vi "Request Events FG.vi"(7 "Action (Get)":enum16{"Initialize", "Get", "Destroy"}(ring)=enum."Get", 8 "error in":errorcluster) -> (0 "error out":errorcluster, 3 "Request Events":T1)   [LabVIEW 2013]
uses:
  Controls_LVTM/RequestEvents.ctl
  Controls_LVTM/UserEventDataPause.ctl
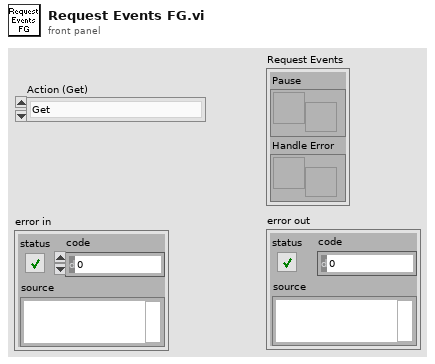
[diagram p1: front panel]
types:
  T1 = typedef "RequestEvents.ctl" = cluster{"Pause":refnum<user-event>, "Handle Error":refnum<user-event>}
  T2 = typedef "UserEventDataPause.ctl" = cluster{"VI":string}
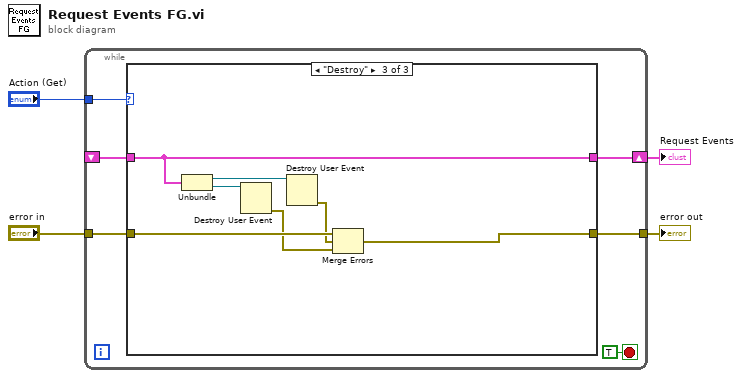
[diagram p0: block diagram]
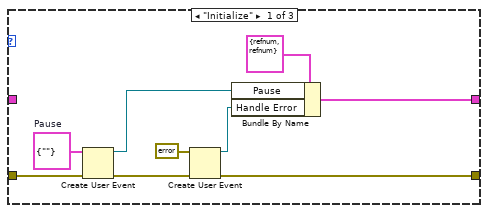
[diagram p2: hidden frame]
diagram:
  n1 = while {
    tunnel: "Action (Get)" -> [w10]
    shift-right: [w7] -> w1
    shift-left: _ -> [w6]
    tunnel: "error in" -> [w9]
    tunnel: [w8] -> w2
    stop <- TRUE stop-if-true
    n2 = case shown="\"Destroy\"" w10 {
      tunnel: w9 -> [w16 w20 w28]
      tunnel: [w12 w20 w25] -> w8
      tunnel: [w15 w21 w27] -> w7
      tunnel: w6 -> [_ w21 w27]
      frame "Initialize" {
        w19 = T2 {"VI"=""}  # Pause
        n3 = Create User Event(user event datatype=w19, error in=w16) -> (user event=w17:refnum<user-event>, error out=w11:errorcluster)
        n4 = Create User Event(user event datatype=errorcluster {"status"=FALSE, "code"=0, "source"=""} ("Error"), error in=w11) -> (user event=w13:refnum<user-event>, error out=w12:errorcluster)
        n5 = Bundle By Name(cluster=T1 {"Pause"=refnum, "Handle Error"=refnum}, "Pause"=w17, "Handle Error"=w13) -> (w15:T1)
      }
      frame "Get" {
      }
      frame "Destroy" {
        n6 = Unbundle(w27) -> ("Pause"=w26:refnum<user-event>, "Handle Error"=w23:refnum<user-event>)
        n7 = Destroy User Event(user event=w23) -> (error out=w22:errorcluster)  [unwired: 1 in]
        n8 = Destroy User Event(user event=w26) -> (error out=w24:errorcluster)  [unwired: 1 in]
        n9 = Merge Errors(w28, w24, w22) -> (w25:errorcluster)
      }
    }
  }
  "error out" <- w2
  "Request Events" <- w1
